vi "WPI_AccumulatorInit.vi"(8 "error in (no error)":errorcluster, 11 "AIDeviceRef":T1={"DevStatus"={"status"=FALSE, "code"=0, "source"=""}, "Analog Channel"=enum."Invalid"}) -> (0 "error out":errorcluster, 3 "AIDeviceRef":T1={"DevStatus"={"status"=FALSE, "code"=0, "source"=""}, "Analog Channel"=enum."Invalid"})   [LabVIEW 2017]
doc: "Initializes the accumulator on the FPGA on the CompactRIO device. Initializing the accumulator sets the center value of the accumulator to zero and sets the cumulative accumulator value to zero."
uses:
  <vilib>/Rock Robotics/WPI/AnalogChannel/WPI_AnalogChannelDevRef.ctl
  <vilib>/Rock Robotics/SystemInterfaces/AI/FPGA_AIChannel.ctl
  <vilib>/Rock Robotics/SystemInterfaces/System/FPGA_SystemGet.vi
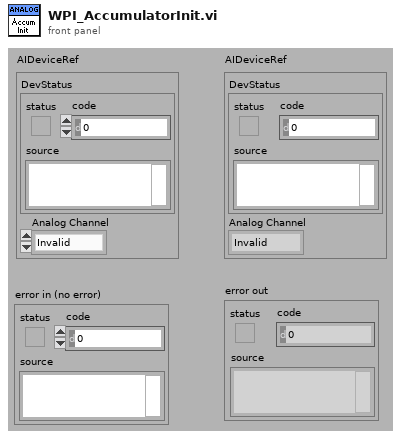
[diagram p1: front panel]
types:
  T1 = typedef "WPI_AnalogChannelDevRef.ctl" = cluster{"DevStatus":errorcluster, "Analog Channel":T2}
  T2 = typedef "FPGA_AIChannel.ctl" = enum8{"AI 0", "AI 1", "AI 2", "AI 3", "AI MXP 0", "AI MXP 1", "AI MXP 2", "AI MXP 3", "Invalid"}
  T3 = typedef "FPGA_AIDevRef.ctl" = cluster{"DevStatus":errorcluster}
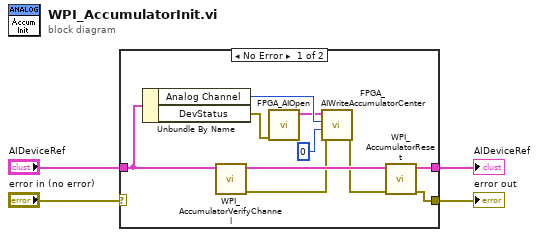
[diagram p0: block diagram]
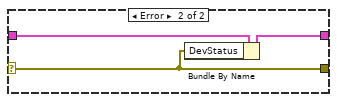
[diagram p2: hidden frame]
diagram:
  n1 = case shown="No Error" "error in (no error)" {
    selector: "error in (no error)" -> [_ w15]
    tunnel: [w14 w16] -> w4
    tunnel: [w13 w15] -> w3
    tunnel: "AIDeviceRef" -> [w8 w17]
    frame No Error {
      n2 = Unbundle By Name(w8) -> ("Analog Channel"=w12:T2, "DevStatus"=w10:errorcluster)
      n3 = call <vilib>:"WPI_AccumulatorVerifyChannel.vi"("AIDeviceRef"=w8) -> ("error out"=w6:errorcluster, "AIDeviceRef"=w7:T1)  [unwired: 9 in]
      n4 = call <vilib>:"FPGA_AIOpen.vi"("error in (no error)"=w10) -> ("AI Reference out"=w11:T3)  [unwired: 2 in, 8 out]
      n5 = call <vilib>:"FPGA_AIWriteAccumulatorCenter.vi"("error in (no error)"=w6, "Center"=0, "Channel"=w12, "AI Reference in"=w11) -> ("error out"=w5:errorcluster)  [unwired: 7 out]
      n6 = call <vilib>:"WPI_AccumulatorReset.vi"("error in (no error)"=w5, "AIDeviceRef"=w7) -> ("error out"=w13:errorcluster, "AIDeviceRef"=w14:T1)  [unwired: 8 out]
    }
    frame Error {
      n7 = Bundle By Name(cluster=w17, "DevStatus"=w15) -> (w16:T1)
    }
  }
  "AIDeviceRef" <- w4
  "error out" <- w3
